vi "cylinder 1.vi"(10 "Element value":dbl, 11 "Boolean":bool) -> (1 "Element 3":dbl, 2 "Element 2":dbl, 3 "Element 1":dbl)   [LabVIEW 2025]
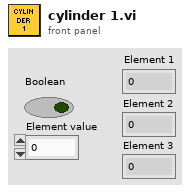
[diagram p1: front panel]
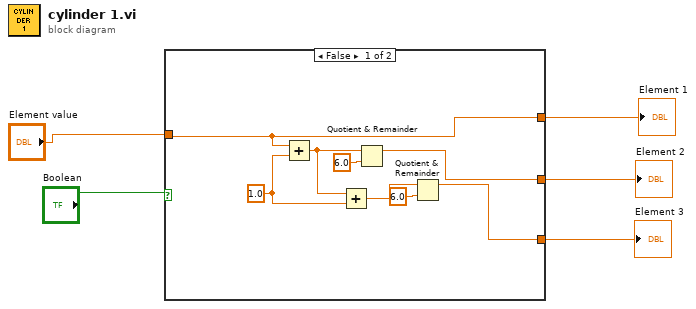
[diagram p0: block diagram]
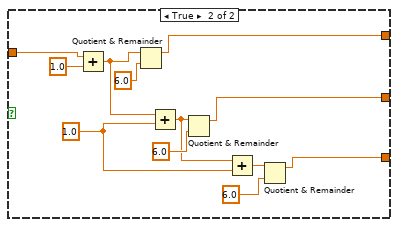
[diagram p2: hidden frame]
diagram:
  n1 = case shown="False" "Boolean" {
    tunnel: [w10 w17] -> w5
    tunnel: [w9 w16] -> w4
    tunnel: [w8 w15] -> w3
    tunnel: "Element value" -> [w10 w14]
    frame False {
      w6 = 1.0 ("y")
      n2 = Add(x=w10, y=w6) -> (x+y=w7:dbl)
      n3 = Add(x=w7, y=w6) -> (x+y=w13:dbl)
      n4 = Quotient & Remainder(x=w7, y=6.0) -> (x-y*floor(x/y)=w9:dbl)  [unwired: 1 out]
      n5 = Quotient & Remainder(x=w13, y=6.0) -> (x-y*floor(x/y)=w8:dbl)  [unwired: 1 out]
    }
    frame True {
      w24 = 1.0 ("y")
      n6 = Add(x=w14, y=1.0) -> (x+y=w20:dbl)
      n7 = Quotient & Remainder(x=w20, y=6.0) -> (x-y*floor(x/y)=w17:dbl)  [unwired: 1 out]
      n8 = Add(x=w20, y=w24) -> (x+y=w18:dbl)
      n9 = Quotient & Remainder(x=w18, y=6.0) -> (x-y*floor(x/y)=w16:dbl)  [unwired: 1 out]
      n10 = Add(x=w18, y=w24) -> (x+y=w23:dbl)
      n11 = Quotient & Remainder(x=w23, y=6.0) -> (x-y*floor(x/y)=w15:dbl)  [unwired: 1 out]
    }
  }
  "Element 1" <- w5
  "Element 2" <- w4
  "Element 3" <- w3
